vi "Constructor.vi"(10 "Capacity":u32) -> (3 "TypedCircularBuffer out":refnum<class "RefTypedCircularBuffer.lvclass">)   [LabVIEW 2024, in "RefTypedCircularBuffer.lvclass"]
uses:
  RefTypedCircularBuffer.lvclass
  RefTypedCircularBuffer.lvclass/RefTypedCircularBuffer.ctl
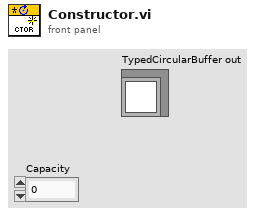
[diagram p1: front panel]
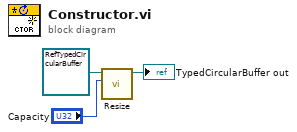
[diagram p0: block diagram]
diagram:
  n1 = call "Resize.vi"("Capacity"="Capacity", "TypedCircularBuffer in"=refnum<class "RefTypedCircularBuffer.lvclass"> refnum ("TypedCircularBuffer.lvclass")) -> ("TypedCircularBuffer out"=→"TypedCircularBuffer out":refnum<class "RefTypedCircularBuffer.lvclass">)  [unwired: 9 in]
